vi "workbook new.vi"(8 "error in (no error)":errorcluster, 11 "filename":string) -> (0 "error out":errorcluster, 3 "function return":u32)   [LabVIEW 2015, in "xlsxwriter.lvlib"]
doc: "lxw_workbook workbook_new(const char *filename);"
uses:
  xlsxwriter.lvlib
  xlsxwriter.dll
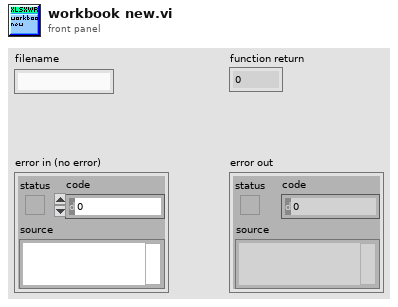
[diagram p1: front panel]
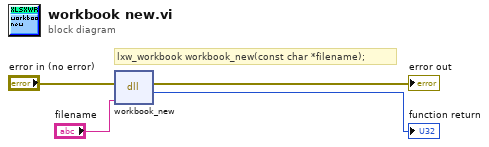
[diagram p0: block diagram]
diagram:
  # "lxw_workbook workbook_new(const char *filename);"
  n1 = dll-call lib="C:/Users/WDAGUtilityAccount/Desktop/lv_vis_added_cell/xlsxwriter.*" fn="workbook_new"(error in="error in (no error)", "filename"="filename") -> (error out=→"error out":errorcluster, →"function return":u32)  [unwired: 3 in, 1 out]
